vi "query_UIM_MCFG.vi"(8 "error in (no error)":errorcluster caption="错误输入（无错误）", 11 "StepMotor输入":refnum<class "StepMotor.lvclass">) -> (0 "error out":errorcluster caption="错误输出", 2 "MCFG输入":T1, 3 "StepMotor输出":refnum<class "StepMotor.lvclass">)   [LabVIEW 2016, in "MotionControl.lvlib" / "StepMotor.lvclass"]
uses:
  <userlib>/MotionControl/StepMotor/StepMotor.lvclass
  <userlib>/MotionControl/StepMotor/StepMotor.lvclass/StepMotor.ctl
  <userlib>/UISimCanFunc_wrapper/UISimCanFunc_wrapper.lvlib
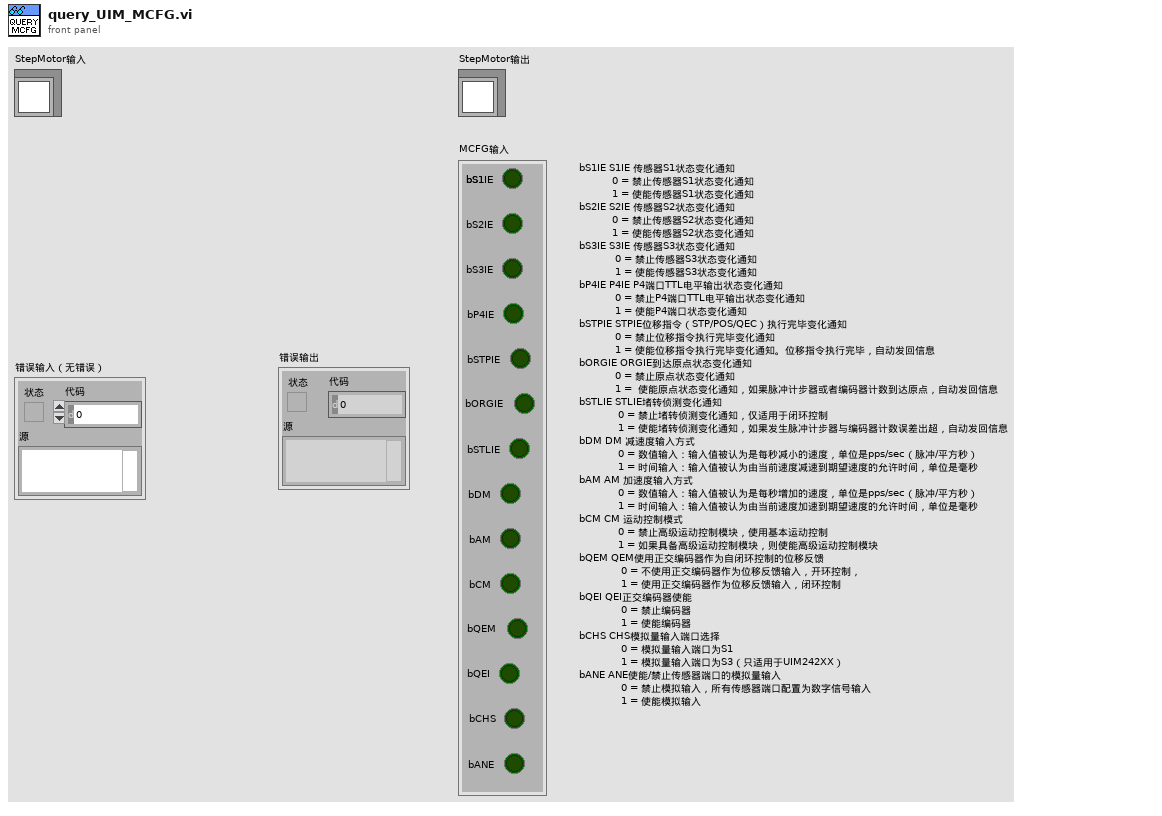
[diagram p1: front panel]
types:
  T1 = cluster{"bS1IE":bool, "bS2IE":bool, "bS3IE":bool, "bP4IE":bool, "bSTPIE":bool, "bORGIE":bool, "bSTLIE":bool, "bDM":bool, "bAM":bool, "bCM":bool, "bQEM":bool, "bQEI":bool, "bCHS":bool, "bANE":bool}
  T2 = typedef "UISimCanFunc_wrapper.lvlib/UIM_MCFG_INFO_OBJ.ctl" = cluster{" bS1IE":bool, " bS2IE":bool, " bS3IE":bool, " bP4IE":bool, " bSTPIE":bool, " bORGIE":bool, " bSTLIE":bool, " bDM":bool, " bAM":bool, " bCM":bool, " bQEM":bool, " bQEI        ":bool, " bCHS":bool, " bANE":bool}
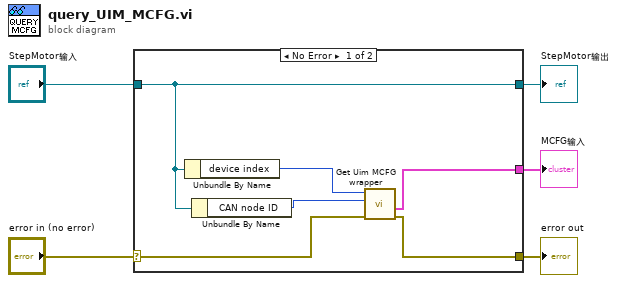
[diagram p0: block diagram]
diagram:
  n1 = case shown="No Error" "error in (no error)" {
    selector: "error in (no error)" -> [w8 w12]
    tunnel: [w7 w12] -> w4
    tunnel: [w11 w13] -> w2
    tunnel: "StepMotor输入" -> [w11 w13]
    tunnel: [w6 _] -> w1
    frame No Error {
      n2 = Unbundle By Name(w11) -> ("device index"=w10:u32)
      n3 = Unbundle By Name(w11) -> ("CAN node ID"=w9:u32)
      n4 = call <userlib>:"Get Uim MCFG wrapper.vi"("error in (no error)"=w8, "dwCanNodeId"=w9, "dwDevIndex"=w10) -> ("error out"=w7:errorcluster, "UIM_MCFG_INFO_OBJ"=w6:T2)  [unwired: 6 in, 1 out]
    }
    frame Error {
    }
  }
  "error out" <- w4
  "StepMotor输出" <- w2
  "MCFG输入" <- w1
